vi "采配水仪器参数改变发送 (子VI).vi"(8 "错误输入":errorcluster caption="错误输出") -> (0 "错误输出":errorcluster)   [LabVIEW 2016, in "数据传输系统-03.lvlib"]
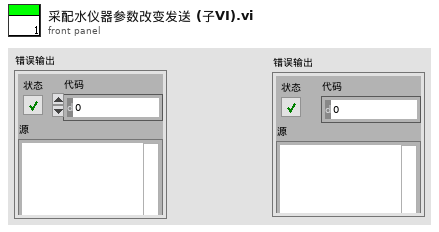
[diagram p1: front panel]
types:
  T1 = cluster{"CODMn关键参数":bool, "氨氮关键参数":bool, "总磷关键参数":bool, "总氮关键参数":bool, "CODCr关键参数":bool, "采配水关键参数":bool}
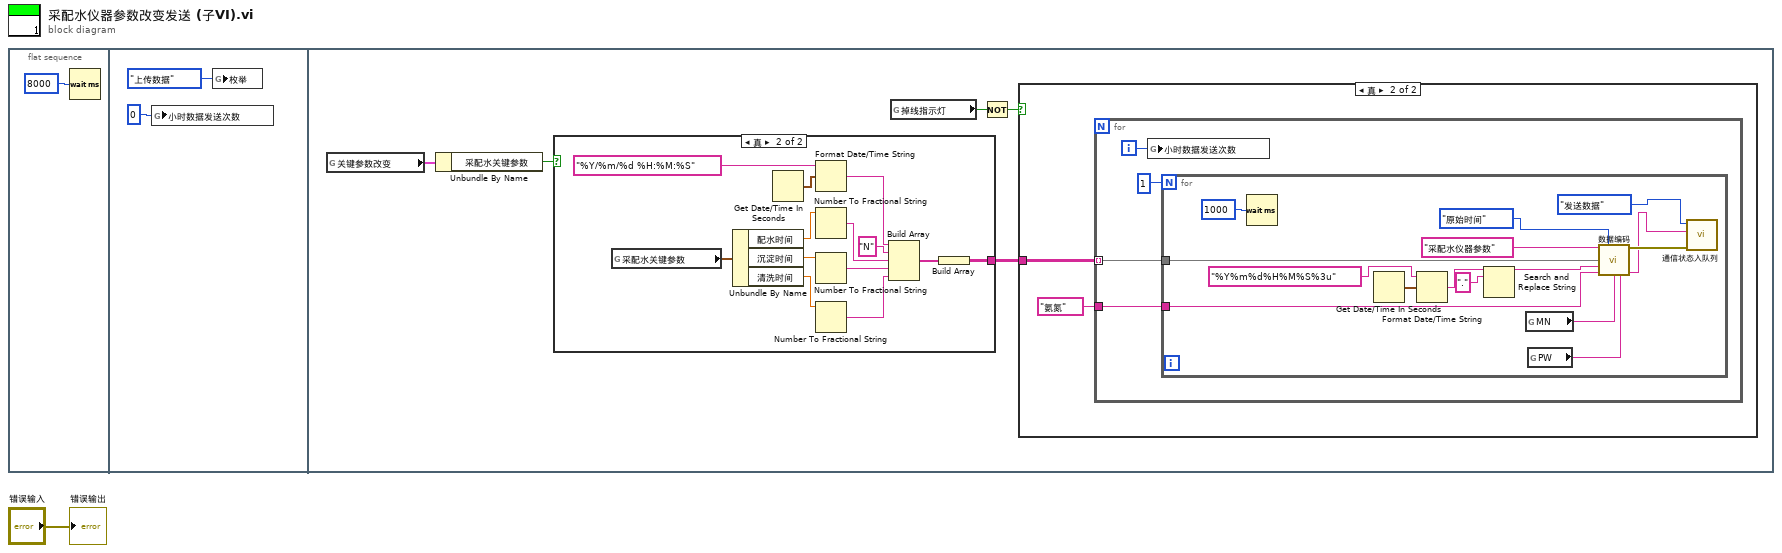
[diagram p0: block diagram]
diagram:
  n1 = flat-sequence {
    frame #0 {
      n2 = Wait (ms)(milliseconds to wait=u32 8000 ("等待时间（毫秒）")) -> ()  [unwired: 1 out]
    }
    frame #1 {
      n3 = global write "全局 小时数据发送次数.vi" "小时数据发送次数"(0 ("小时数据发送次数")) -> ()
      n4 = global write "全局1.vi" "枚举"(enum16{"返回请求应答", "上传数据", "返回执行结果"}."上传数据" ("枚举")) -> ()
    }
    frame #2 {
      n5 = global read "全局1.vi" "关键参数改变"() -> (w7:T1)
      n6 = Unbundle By Name(w7) -> ("采配水关键参数"=w6:bool)
      n7 = case shown="真" w6 {
        tunnel: [_ w10] -> w5
        frame False {
        }
        frame True {
          n8 = global read "全局1.vi" "采配水关键参数"() -> (w22:cluster{"配水时间":dbl, "沉淀时间":dbl, "清洗时间":dbl})
          n9 = Unbundle By Name(w22) -> ("配水时间"=w21:dbl, "沉淀时间"=w20:dbl, "清洗时间"=w19:dbl)
          n10 = Get Date/Time In Seconds() -> (seconds since 1Jan1904=w13:timestamp)
          n11 = Format Date/Time String(time format string (%c)="%Y/%m/%d %H:%M:%S" ("时间格式字符串(%c)"), seconds (now)=w13) -> (date/time string=w11:string)  [unwired: 1 in]
          n12 = Number To Fractional String(number=w21) -> (F-format string=w17:string)  [unwired: 3 in]
          n13 = Number To Fractional String(number=w20) -> (F-format string=w16:string)  [unwired: 3 in]
          n14 = Number To Fractional String(number=w19) -> (F-format string=w15:string)  [unwired: 3 in]
          n15 = Build Array(w11, "N", w17, w16, w15) -> (w18:string[])
          n16 = Build Array(w18) -> (w10:string[][])
        }
      }
      n17 = global read "全局 数据发送重叠.vi" "掉线指示灯"() -> (w9:bool)
      n18 = Not(x=w9) -> (.not. x?=w8:bool)
      n19 = case shown="真" w8 {
        tunnel: w5 -> [_ w23]
        frame False {
        }
        frame True {
          n20 = for {
            tunnel: "氨氮" ("污染物编码") -> [w28]
            tunnel: w23 -> [w27] mode=indexing
            i -> [w26]
            n21 = global write "全局 小时数据发送次数.vi" "小时数据发送次数"(w26) -> ()
            n22 = for {
              N: 1 -> [_]
              tunnel: w28 -> [w34]
              tunnel: w27 -> [w33]
              n23 = Wait (ms)(milliseconds to wait=u32 1000 ("等待时间（毫秒）")) -> ()  [unwired: 1 out]
              n24 = Get Date/Time In Seconds() -> (seconds since 1Jan1904=w41:timestamp)
              n25 = Format Date/Time String(time format string (%c)="%Y%m%d%H%M%S%3u" ("时间格式字符串(%c)"), seconds (now)=w41) -> (date/time string=w40:string)  [unwired: 1 in]
              n26 = Search and Replace String(input string=w40, search string="." ("搜索字符串")) -> (result string=w38:string)  [unwired: 6 in, 3 out]
              n27 = global read "断电保存全局.vi" "MN"() -> (w37:string)
              n28 = global read "断电保存全局.vi" "PW"() -> (w36:string)
              n29 = call "数据编码.vi"("table输入"="采配水仪器参数" ("新元素/子数组"), "仪器参数上传时间"=enum16{"精确到小时", "原始时间"}."原始时间", "仪器参数"=w33, "QN"=w38, "参数"=w34, "MN"=w37, "PW"=w36) -> ("错误常量"=w35:errorcluster, "通讯包字符串"=w29:string)  [unwired: 7 in]
              n30 = call "通信状态入队列.vi"("错误输入（无错误）"=w35, "发送报文"=w29, "枚举"=enum16{"打开连接", "发送数据", "读取数据", "数据处理", "关闭连接"}."发送数据") -> ()  [unwired: 8 in, 1 out]
            }
          }
        }
      }
    }
  }
  "错误输出" <- "错误输入"
